vi "Get VI By Folder Expand.vi"(8 "error in (no error)":errorcluster {"code" format="Error %.0f"}, 11 "VIDoc Printer - Confluence In":refnum<class "VIDoc Printer - Confluence.lvclass">) -> (0 "error out":errorcluster {"code" format="Error %.0f"}, 2 "By Folder Expand":bool=TRUE, 3 "VIDoc Printer - Confluence Out":refnum<class "VIDoc Printer - Confluence.lvclass">)   [LabVIEW 2023, in "VIDoc Printer - Confluence.lvlib" / "VIDoc Printer - Confluence.lvclass"]
uses:
  VIDoc Printer - Confluence.lvclass
  VIDoc Printer - Confluence.lvclass/VIDoc Printer - Confluence.ctl
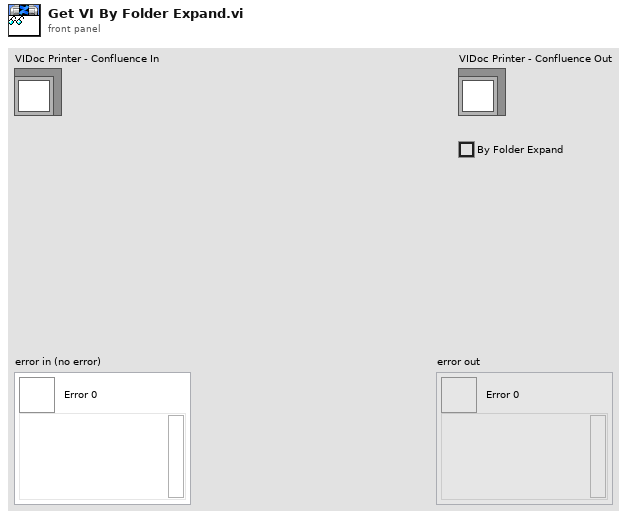
[diagram p1: front panel]
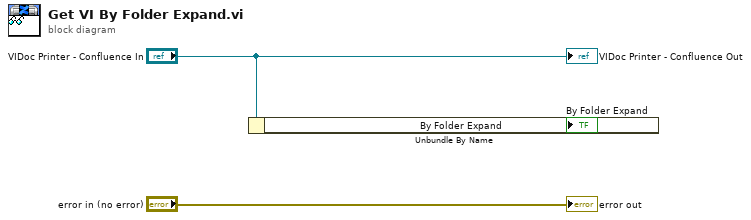
[diagram p0: block diagram]
diagram:
  n1 = Unbundle By Name("VIDoc Printer - Confluence In") -> ("By Folder Expand"=→"By Folder Expand":bool)
  "error out" <- "error in (no error)"
  "VIDoc Printer - Confluence Out" <- "VIDoc Printer - Confluence In"
